vi "timer1.vi"(11 "reset":bool) -> (3 "Numeric":dbl)   [LabVIEW 2019]
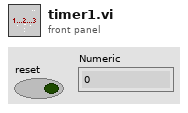
[diagram p1: front panel]
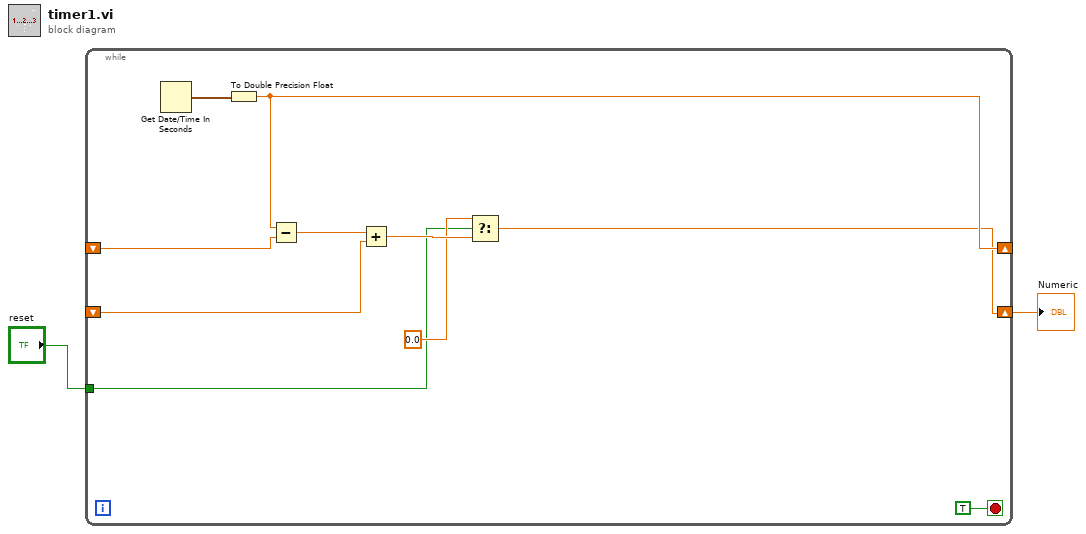
[diagram p0: block diagram]
diagram:
  n1 = while {
    shift-right: [w11] -> _
    shift-left: _ -> [w12]
    shift-right: [w6] -> w1
    shift-left: _ -> [w4]
    tunnel: "reset" -> [w5]
    stop <- TRUE stop-if-true
    n2 = Get Date/Time In Seconds() -> (seconds since 1Jan1904=w3:timestamp)
    n3 = To Double Precision Float(number=w3) -> (double precision float=w11:dbl)
    n4 = Subtract(x=w11, y=w12) -> (x-y=w10:dbl)
    n5 = Add(x=w10, y=w4) -> (x+y=w8:dbl)
    n6 = Select(t=0.0, s=w5, f=w8) -> (s? t:f=w6:dbl)
  }
  "Numeric" <- w1
